vi "WriteProps.vi"(2 "Bands":T1, 8 "error in (no error)":errorcluster, 11 "StateFunction in":refnum<class "StateFunction.lvclass">) -> (0 "error out":errorcluster, 3 "StateFunction out":refnum<class "StateFunction.lvclass">)   [LabVIEW 2014, in "StateFunction.lvclass"]
uses:
  StateFunction.lvclass
  Typedef/ChannelProperties.ctl
panel:
  # "Band"
  # "frequency (Hz)"
  # "phase (deg)"
  # "index"
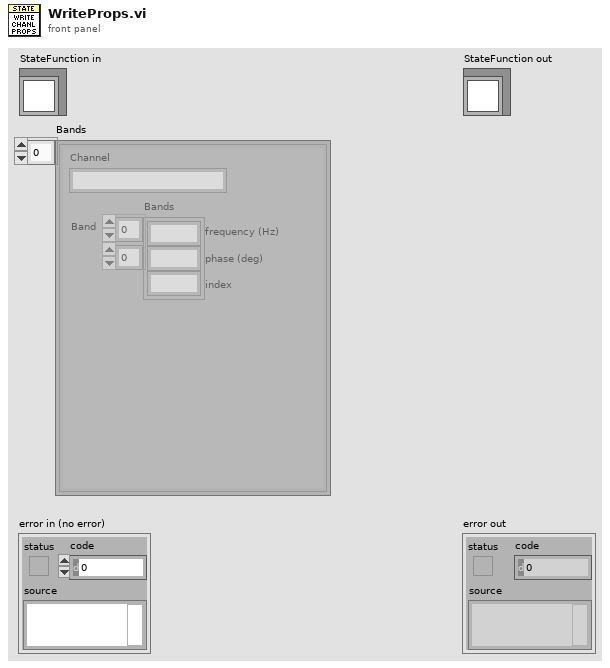
[diagram p1: front panel]
types:
  T1 = typedef "StateFunction.lvclass/ChannelProperties.ctl" = cluster{"Channel":string, "Bands":dbl[][]}[]
  T2 = typedef "Functions.lvlib/ArbitraryFunction.lvclass/Arbitrary.ctl" = cluster{"Handle":string, "Size":i32, "Gain":dbl, "Offset":dbl, "Waveform":waveform(dbl)}
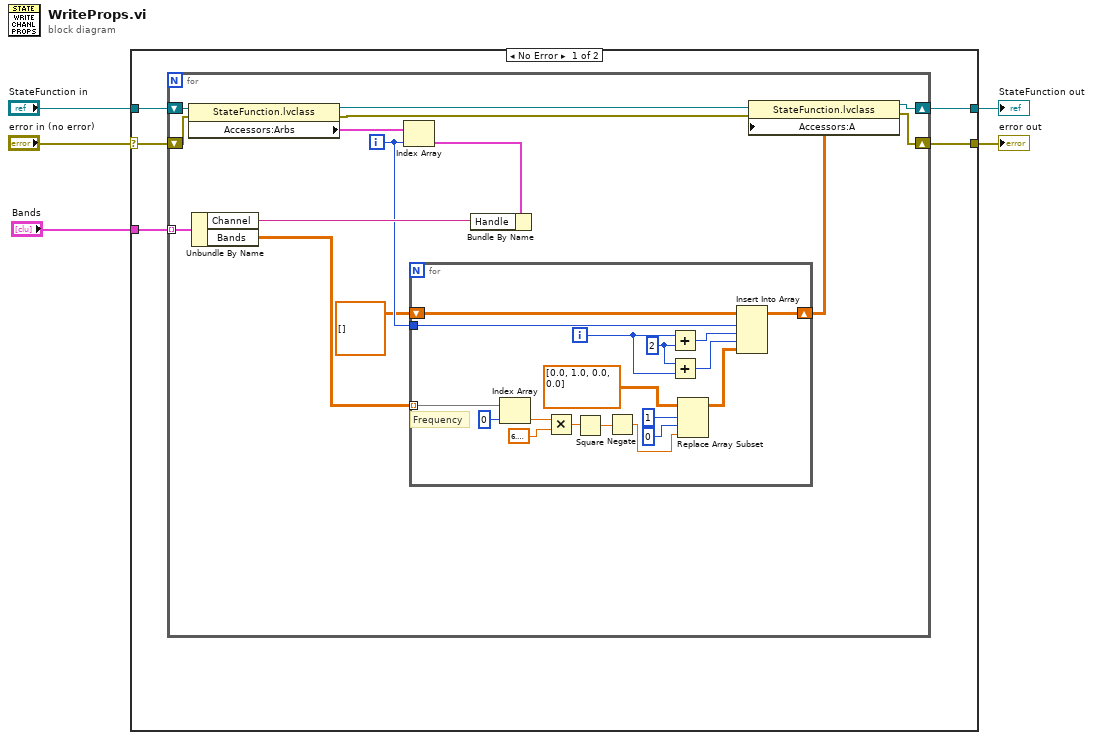
[diagram p0: block diagram]
diagram:
  n1 = case shown="No Error" "error in (no error)" {
    selector: "error in (no error)" -> [w8 w44]
    tunnel: [w6 w44] -> w4
    tunnel: [w7 w43] -> w2
    tunnel: "StateFunction in" -> [w9 w43]
    tunnel: "Bands" -> [w10 _]
    frame No Error {
      n2 = for {
        tunnel: w10 -> [w24] mode=indexing
        shift-right: [w11] -> w7
        shift-left: w9 -> [w23]
        shift-right: [w12] -> w6
        shift-left: w8 -> [w19]
        i -> [w17]
        n3 = property class="StateFunction.lvclass"(reference=w23, error in=w19) -> (reference out=w15:refnum<class "StateFunction.lvclass">, error out=w13:errorcluster, "Accessors:Arbs"=w22:T2[])
        n4 = Unbundle By Name(w24) -> ("Channel"=w20:string, "Bands"=w18:dbl[][])
        n5 = Index Array(array=w22, index=w17) -> (element=w21:T2)
        n6 = for {
          tunnel: w18 -> [w42] mode=indexing
          shift-right: [w26] -> w14
          shift-left: dbl[][][] [] ("A") -> [w32]
          tunnel: w17 -> [w30]
          i -> [w29]
          w25 = 2 ("y")
          # "Frequency"
          n7 = Index Array(array=w42, index=0) -> (element=w39:dbl)
          n8 = Multiply(x=w39, y=6.283185307179586) -> (x*y=w37:dbl)
          n9 = Square(x=w37) -> (x^2=w40:dbl)
          n10 = Negate(x=w40) -> (-x=w33:dbl)
          n11 = Add(x=w29, y=w25) -> (x+y=w28:i32)
          n12 = Add(x=w25, y=w29) -> (x+y=w27:i32)
          n13 = Replace Array Subset(array=dbl[][] [[0.0, 1.0], [0.0, 0.0]], new element=w33, index (row)=1, index (col)=0 ("disabled index (col)")) -> (w31:dbl[][])
          n14 = Insert Into Array(array=w32, index (dim 0)=w30, index (dim 1)=w28, index (dim 2)=w27, new element=w31) -> (w26:dbl[][][])
        }
        n15 = Bundle By Name(cluster=w21, "Handle"=w20) -> ()  [unwired: 1 out]
        n16 = property class="StateFunction.lvclass"(reference=w15, error in=w13, "Accessors:A"=w14) -> (reference out=w11:refnum<class "StateFunction.lvclass">, error out=w12:errorcluster)
      }
    }
    frame Error {
    }
  }
  "error out" <- w4
  "StateFunction out" <- w2
